vi "PV HLT5xx Extern pressure sensor.vi"(7 "Adress of unit":u16=1 min=1 max=999 step=1, 8 "error in (no error)":errorcluster, 9 "set extern pressure sensor":u16(ring) items=["intern sensor activ", "extern sensor activ"], 10 "Parameter\nread only<->describe":bool, 11 "VISA session":refnum<visa-resource-name>) -> (0 "error out":errorcluster, 1 "extern pressure sensor out":u16(ring) items=["intern sensor activ", "extern sensor activ"], 2 "response (data)":string, 3 "dup VISA session":refnum<visa-resource-name>)   [LabVIEW 2016, in "Pfeiffer Vacuum.lvlib"]
doc: "This VI allows you to set or check the \"Extern pressure sensor (Para 630)\" on the SmartTest (HLT5xx)."
uses:
  Pfeiffer Vacuum.lvlib
panel:
  # "Extern pressure sensor"
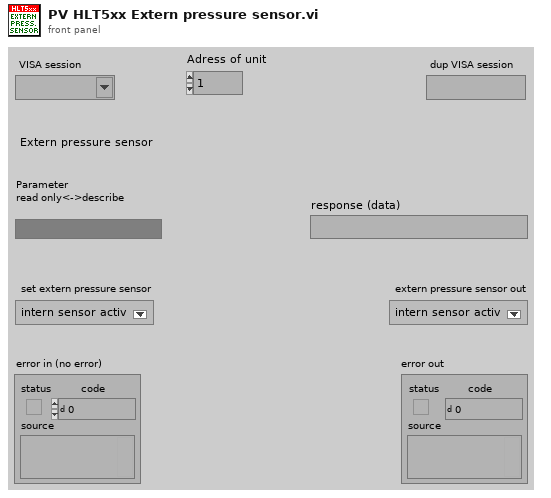
[diagram p1: front panel]
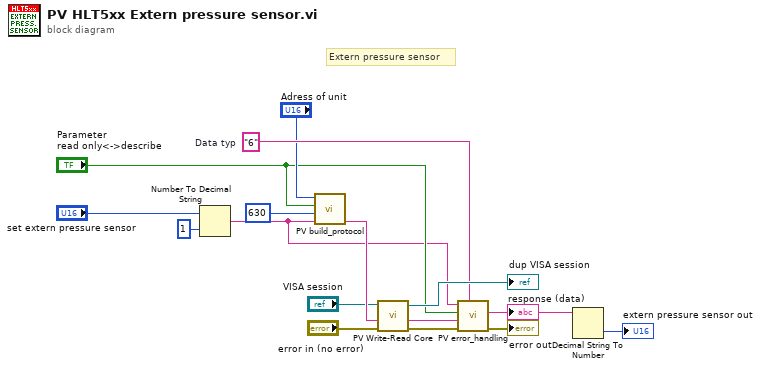
[diagram p0: block diagram]
diagram:
  w11 = "6"  # Data typ
  # "Extern pressure sensor"
  n1 = Number To Decimal String(number="set extern pressure sensor", width (-)=i16 1 ("Breite (-)")) -> (decimal integer string=w3:string)
  n2 = call "PV build_protocol.vi"("Data"=w3, "Parameter-number"=u16 630, "parameter\nread<->describe"="Parameter\nread only<->describe", "Adress"="Adress of unit") -> ("output"=w15:string)  [unwired: 3 in]
  n3 = call "PV Write-Read Core.vi"("error in"="error in (no error)", "Write data in"=w15, "VISA session"="VISA session") -> ("error out"=w13:errorcluster, "response (data) out"=w14:string, "dup VISA session"=→"dup VISA session":refnum<visa-resource-name>)  [unwired: 2 in]
  n4 = call "PV error_handling.vi"("Data Typ in"=w11, "error in"=w13, "response (data) in"=w14, "Parameter\nread only<->describe"="Parameter\nread only<->describe", "data in"=w3) -> ("error out"=→"error out":errorcluster, "Data out"=w9:string)  [unwired: 4 in, 1 out]
  "response (data)" <- w9
  n5 = Decimal String To Number(string=w9) -> (number=→"extern pressure sensor out":i32)  [unwired: 2 in, 1 out]
